vi "Sensor Reads.vi"() -> ()   [LabVIEW 2017]
uses:
  Refnum Names.vi
  <vilib>/Rock Robotics/Network Tables/NT Write Boolean.vi
  Lift/Lift Globals.vi
  <vilib>/Rock Robotics/WPI/ThirdParty/Phoenix-LabVIEW/Motor Controller/Get/CTRE_Phoenix_MotorController_GetSelectedSensorData.vi
  <vilib>/Rock Robotics/Network Tables/NT Write Number.vi
  Intake/Intake Globals.vi
  Intake Rotation/Intake Rotation Globals.vi
  <vilib>/Rock Robotics/WPI/ThirdParty/Phoenix-LabVIEW/Pigeon IMU/CTRE_PigeonIMU_GetRawGyro.vi
  <vilib>/Rock Robotics/WPI/ThirdParty/Phoenix-LabVIEW/Pigeon IMU/CTRE_PigeonIMU_GetYPR.vi
  Drive/Drive Globals.vi
  <vilib>/Rock Robotics/Network Tables/NT Write String.vi
panel:
  out "Z":dbl
  out "Match Time":string
  out "Robot Distance":dbl
  out "Robot Heading":dbl
  out "Arm Position":i32
  out "Cube IR":bool
  out "Arm Upper Limit Switch":bool
  out "Arm Lower Limit Switch":bool
  out "Lift Upper Switch":bool
  out "Lift Lower Switch":bool
  out "Lift Position":i32
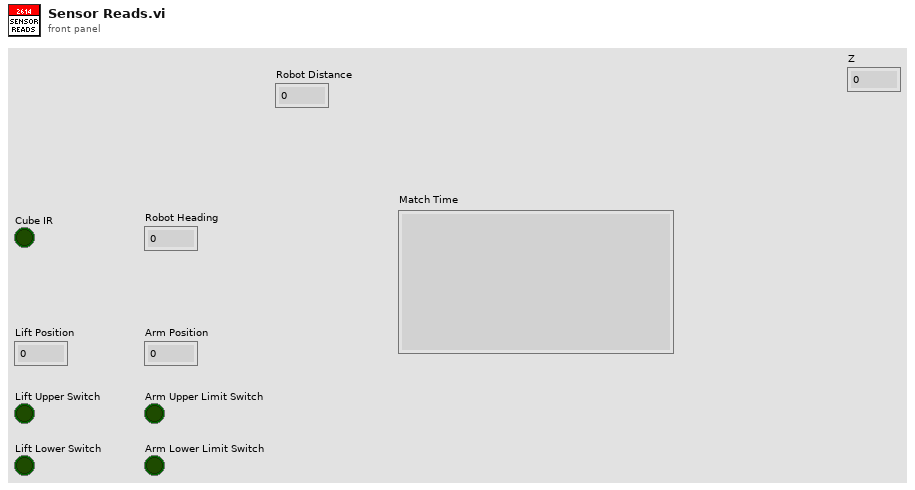
[diagram p1: front panel]
types:
  T1 = typedef "WPI_SwitchDevRef.ctl" = cluster{"DevStatus":errorcluster, "DIO Channel":T2, "CntIndex":T3, "Normally Closed":bool}
  T2 = typedef "FPGA_DIOChannel.ctl" = enum8{"DIO 0", "DIO 1", "DIO 2", "DIO 3", "DIO 4", "DIO 5", "DIO 6", "DIO 7", "DIO 8", "DIO 9", "DIO MXP 0", "DIO MXP 1", "DIO MXP 2", "DIO MXP 3", "DIO MXP 4", "DIO MXP 5", "DIO MXP 6", "DIO MXP 7", "DIO MXP 8", "DIO MXP 9", "DIO MXP 10", "DIO MXP 11", "DIO MXP 12", "DIO MXP 13", "DIO MXP 14", "DIO MXP 15", "SPI Port CS1", "SPI Port CS2", "SPI Port CS3", "SPI Port MISO", "SPI Port MOSI", "Invalid"}
  T3 = typedef "FPGA_CounterCtrSystemIndex.ctl" = enum8{"Ctr 0", "Ctr 1", "Ctr 2", "Ctr 3", "Ctr 4", "Ctr 5", "Ctr 6", "Ctr 7", "Invalid"}
  T4 = typedef "WPI_MotorControlDeviceRef.ctl" = cluster{"DeviceStatus":errorcluster, "Type":T5, "PWM":cluster{"PWM Channel":T6, "DeadBand":T7}, "CAN":cluster{"Device Number":u8, "SetOutput VI Ref":variant, "GetOutput VI Ref":variant, "Enable VI Ref":variant, "Disable VI Ref":variant, "Data":variant}, "Invert":bool, "DIO PWM":cluster{"PWM \"Enable\" Channel":T6, "DIOChannel":T2, "PWM Rate":dbl}}
  T5 = typedef "WPI_MotorControlType.ctl" = enum16{"PWM", "CAN", "DIO PWM"}
  T6 = typedef "FPGA_DIOPWMChannel.ctl" = enum8{"PWM 0", "PWM 1", "PWM 2", "PWM 3", "PWM 4", "PWM 5", "PWM 6", "PWM 7", "PWM 8", "PWM 9", "PWM MXP 0", "PWM MXP 1", "PWM MXP 2", "PWM MXP 3", "PWM MXP 4", "PWM MXP 5", "PWM MXP 6", "PWM MXP 7", "PWM MXP 8", "PWM MXP 9", "Invalid"}
  T7 = typedef "WPI_PWMDeadband.ctl" = cluster{"Name":string, "maxPositivePwm":i32, "minPositivePwm":i32, "centerPwm":i32, "maxNegativePwm":i32, "minNegativePwm":i32, "angularRange":u16}
  T8 = typedef "WPI_DigitalInputDevRef.ctl" = cluster{"DevStatus":errorcluster, "DIO Channel":T2}
  T9 = typedef "CTRE_PigeonIMU_DeviceRef.ctl" = cluster{"DeviceStatus":errorcluster, "Device Number":u8, "Type":T10, "Device ID":u32, "Handle":u64, "UsageFrame":u32, "Library Path":path}
  T10 = typedef "CTRE_PigeonIMU_ConnectionType.ctl" = u32
  T11 = cluster{"X":dbl, "Y":dbl, "Z":dbl, "Magnitude":dbl}
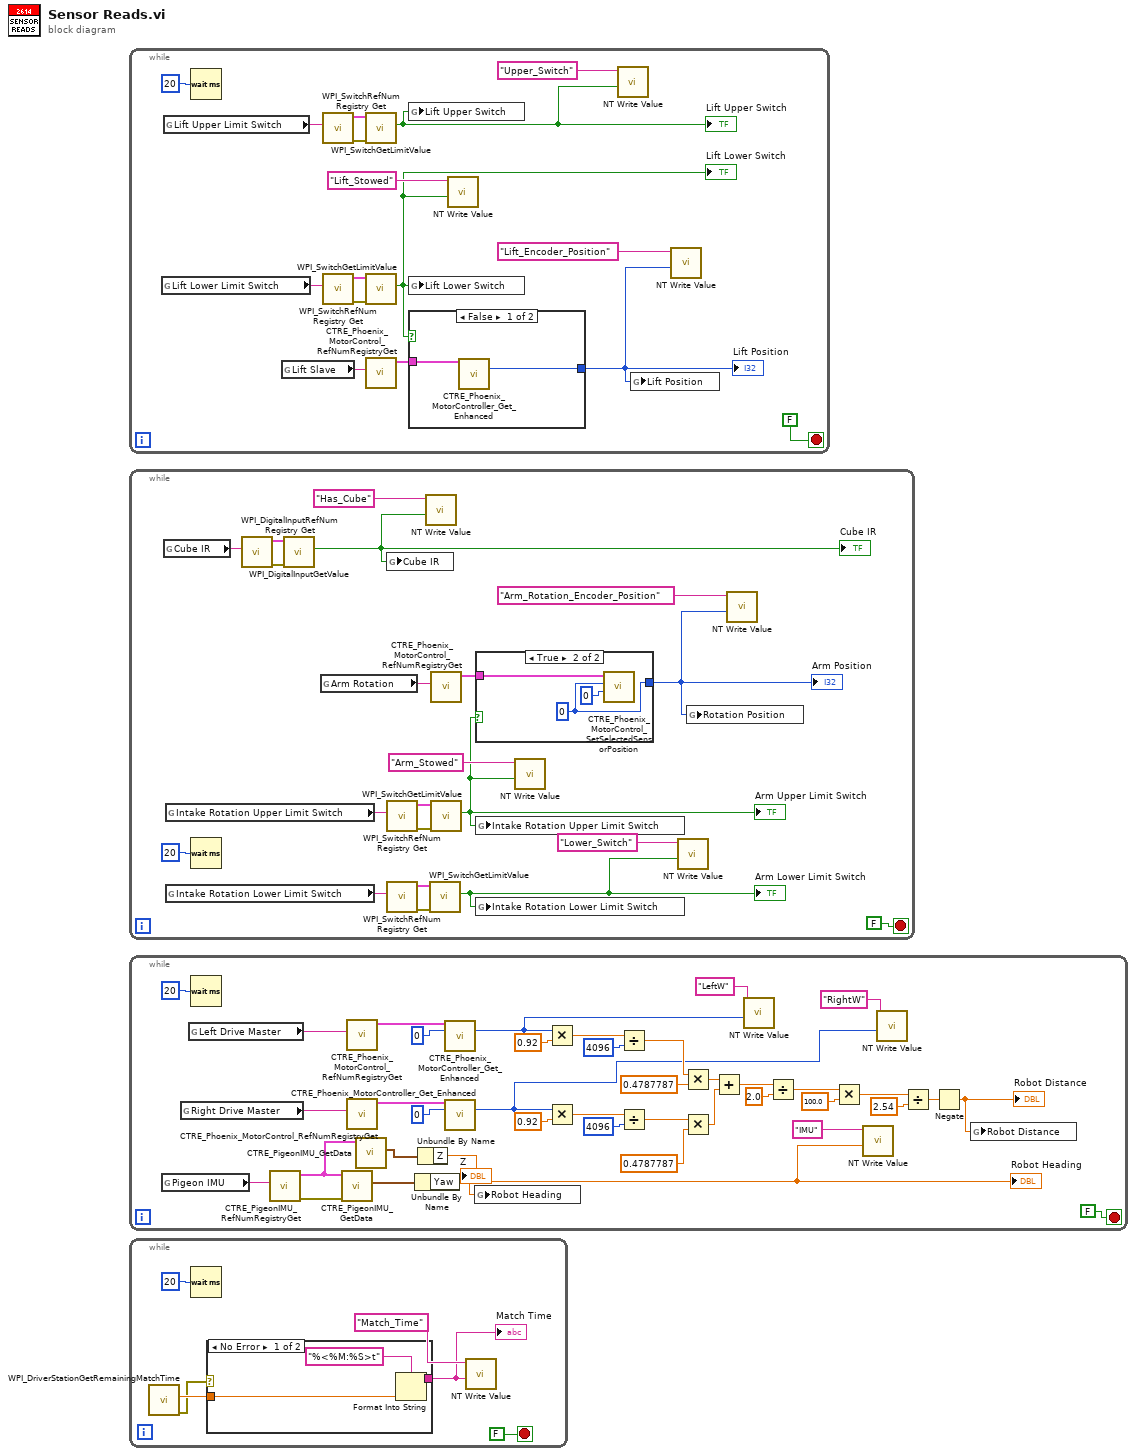
[diagram p0: block diagram]
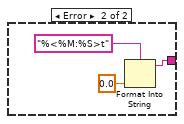
[diagram p2: hidden frame]
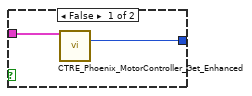
[diagram p3: hidden frame]
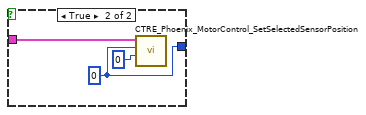
[diagram p4: hidden frame]
diagram:
  n1 = while {
    stop <- FALSE stop-if-true
    n2 = global read "Refnum Names.vi" "Lift Lower Limit Switch"() -> (w11:string)
    n3 = global read "Refnum Names.vi" "Lift Upper Limit Switch"() -> (w12:string)
    n4 = Wait (ms)(milliseconds to wait=u32 20) -> ()  [unwired: 1 out]
    n5 = global read "Refnum Names.vi" "Lift Slave"() -> (w8:string)
    n6 = call <vilib>:"WPI_SwitchRefNum Registry Get.vi"("refnum name"=w12) -> ("error out"=w13:errorcluster, "SwitchDevRef"=w14:T1)  [unwired: 9 in]
    n7 = call <vilib>:"WPI_SwitchRefNum Registry Get.vi"("refnum name"=w11) -> ("error out"=w10:errorcluster, "SwitchDevRef"=w9:T1)  [unwired: 9 in]
    n8 = call <vilib>:"WPI_SwitchGetLimitValue.vi"("error in (no error)"=w13, "SwitchDevRef"=w14) -> ("Switch Pressed"=w2:bool)  [unwired: 7 in, 2 out]
    "Lift Upper Switch" <- w2
    n9 = call <vilib>:"WPI_SwitchGetLimitValue.vi"("error in (no error)"=w10, "SwitchDevRef"=w9) -> ("Switch Pressed"=w5:bool)  [unwired: 7 in, 2 out]
    "Lift Lower Switch" <- w5
    n10 = call <vilib>:"CTRE_Phoenix_MotorControl_RefNumRegistryGet.vi"("refnum name"=w8) -> ("PhoenixMotorControlDevRef"=w7:T4)  [unwired: 9 in, 1 out]
    n11 = global write "Lift Globals.vi" "Lift Upper Switch"(w2) -> ()
    n12 = global write "Lift Globals.vi" "Lift Lower Switch"(w5) -> ()
    n13 = case shown="False" w5 {
      tunnel: w7 -> [w18 w21]
      tunnel: [w17 w19] -> w3
      frame False {
        n14 = call-poly <vilib>:"CTRE_Phoenix_MotorController_Get_Enhanced.vi"("PhoenixMotorControlDevRef"=w18) -> ("Position (Raw Sensor Units)"=w17:i32)  [unwired: 11 in, 3 out]
      }
      frame True {
        w19 = 0 ("New Sensor Position")
        n15 = call <vilib>:"CTRE_Phoenix_MotorControl_SetSelectedSensorPosition.vi"("pidLoopIdx"=u32 0, "New Sensor Position"=w19, "PhoenixMotorControlDevRef"=w21) -> ()  [unwired: 7 in, 2 out]
      }
    }
    "Lift Position" <- w3
    n16 = call-poly <vilib>:"NT Write Value.vi"("Boolean"=w5, "Name"="Lift_Stowed") -> ()  [unwired: 9 in, 1 out]
    n17 = call-poly <vilib>:"NT Write Value.vi"("Boolean"=w2, "Name"="Upper_Switch") -> ()  [unwired: 9 in, 1 out]
    n18 = global write "Lift Globals.vi" "Lift Position"(w3) -> ()
    n19 = call-poly <vilib>:"NT Write Value.vi"("Numeric"=w3, "Name"="Lift_Encoder_Position") -> ()  [unwired: 9 in, 1 out]
  }
  n20 = while {
    stop <- FALSE stop-if-true
    n21 = global read "Refnum Names.vi" "Cube IR"() -> (w40:string)
    n22 = global read "Refnum Names.vi" "Intake Rotation Upper Limit Switch"() -> (w37:string)
    n23 = global read "Refnum Names.vi" "Intake Rotation Lower Limit Switch"() -> (w36:string)
    n24 = Wait (ms)(milliseconds to wait=u32 20) -> ()  [unwired: 1 out]
    n25 = call <vilib>:"WPI_DigitalInputRefNum Registry Get.vi"("refnum name"=w40) -> ("error out"=w39:errorcluster, "DigitalInputDevRef"=w38:T8)  [unwired: 9 in]
    n26 = call <vilib>:"WPI_DigitalInputGetValue.vi"("error in (no error)"=w39, "DigitalInputDevRef"=w38) -> ("Value"=w26:bool)  [unwired: 7 in, 2 out]
    "Cube IR" <- w26
    n27 = global read "Refnum Names.vi" "Arm Rotation"() -> (w31:string)
    n28 = global write "Intake Globals.vi" "Cube IR"(w26) -> ()
    n29 = call <vilib>:"WPI_SwitchRefNum Registry Get.vi"("refnum name"=w37) -> ("error out"=w33:errorcluster, "SwitchDevRef"=w32:T1)  [unwired: 9 in]
    n30 = call <vilib>:"WPI_SwitchRefNum Registry Get.vi"("refnum name"=w36) -> ("error out"=w34:errorcluster, "SwitchDevRef"=w35:T1)  [unwired: 9 in]
    n31 = call-poly <vilib>:"NT Write Value.vi"("Boolean"=w26, "Name"="Has_Cube") -> ()  [unwired: 9 in, 1 out]
    n32 = call <vilib>:"WPI_SwitchGetLimitValue.vi"("error in (no error)"=w34, "SwitchDevRef"=w35) -> ("Switch Pressed"=w23:bool)  [unwired: 7 in, 2 out]
    "Arm Lower Limit Switch" <- w23
    n33 = call <vilib>:"CTRE_Phoenix_MotorControl_RefNumRegistryGet.vi"("refnum name"=w31) -> ("PhoenixMotorControlDevRef"=w30:T4)  [unwired: 9 in, 1 out]
    n34 = call <vilib>:"WPI_SwitchGetLimitValue.vi"("error in (no error)"=w33, "SwitchDevRef"=w32) -> ("Switch Pressed"=w24:bool)  [unwired: 7 in, 2 out]
    "Arm Upper Limit Switch" <- w24
    n35 = case shown="True" w24 {
      tunnel: [w44 w46] -> w27
      tunnel: w30 -> [w43 w45]
      frame False {
        n36 = call-poly <vilib>:"CTRE_Phoenix_MotorController_Get_Enhanced.vi"("PhoenixMotorControlDevRef"=w43) -> ("Position (Raw Sensor Units)"=w44:i32)  [unwired: 11 in, 3 out]
      }
      frame True {
        w46 = 0 ("New Sensor Position")
        n37 = call <vilib>:"CTRE_Phoenix_MotorControl_SetSelectedSensorPosition.vi"("pidLoopIdx"=u32 0, "New Sensor Position"=w46, "PhoenixMotorControlDevRef"=w45) -> ()  [unwired: 7 in, 2 out]
      }
    }
    "Arm Position" <- w27
    n38 = global write "Intake Rotation Globals.vi" "Intake Rotation Upper Limit Switch"(w24) -> ()
    n39 = global write "Intake Rotation Globals.vi" "Intake Rotation Lower Limit Switch"(w23) -> ()
    n40 = call-poly <vilib>:"NT Write Value.vi"("Boolean"=w24, "Name"="Arm_Stowed") -> ()  [unwired: 9 in, 1 out]
    n41 = call-poly <vilib>:"NT Write Value.vi"("Boolean"=w23, "Name"="Lower_Switch") -> ()  [unwired: 9 in, 1 out]
    n42 = global write "Intake Rotation Globals.vi" "Rotation Position"(w27) -> ()
    n43 = call-poly <vilib>:"NT Write Value.vi"("Numeric"=w27, "Name"="Arm_Rotation_Encoder_Position") -> ()  [unwired: 9 in, 1 out]
  }
  n44 = while {
    stop <- FALSE stop-if-true
    n45 = global read "Refnum Names.vi" "Pigeon IMU"() -> (w85:string)
    n46 = global read "Refnum Names.vi" "Right Drive Master"() -> (w82:string)
    n47 = global read "Refnum Names.vi" "Left Drive Master"() -> (w81:string)
    n48 = Wait (ms)(milliseconds to wait=u32 20) -> ()  [unwired: 1 out]
    n49 = call <vilib>:"CTRE_PigeonIMU_RefNumRegistryGet.vi"("refnum name"=w85) -> ("error out"=w84:errorcluster, "PigeonIMUDevRef"=w49:T9)  [unwired: 9 in]
    n50 = call-poly <vilib>:"CTRE_PigeonIMU_GetData.vi"("error in (no error)"=w84, "PigeonIMUDevRef"=w49) -> ("Yaw Pitch Roll"=w83:cluster{"Yaw":dbl, "Pitch":dbl, "Roll":dbl})  [unwired: 7 in, 2 out]
    n51 = call <vilib>:"CTRE_Phoenix_MotorControl_RefNumRegistryGet.vi"("refnum name"=w81) -> ("PhoenixMotorControlDevRef"=w77:T4)  [unwired: 9 in, 1 out]
    n52 = call <vilib>:"CTRE_Phoenix_MotorControl_RefNumRegistryGet.vi"("refnum name"=w82) -> ("PhoenixMotorControlDevRef"=w80:T4)  [unwired: 9 in, 1 out]
    n53 = call-poly <vilib>:"CTRE_PigeonIMU_GetData.vi"("PigeonIMUDevRef"=w49) -> ("Gyro DPS"=w50:T11)  [unwired: 8 in, 2 out]
    n54 = Unbundle By Name(w83) -> ("Yaw"=w51:dbl)
    "Robot Heading" <- w51
    n55 = Unbundle By Name(w50) -> ("Z"=→"Z":dbl)
    n56 = call-poly <vilib>:"CTRE_Phoenix_MotorController_Get_Enhanced.vi"("PhoenixMotorControlDevRef"=w77, "pidLoopIdx"=u32 0) -> ("Position (Raw Sensor Units)"=w55:i32)  [unwired: 10 in, 3 out]
    n57 = call-poly <vilib>:"CTRE_Phoenix_MotorController_Get_Enhanced.vi"("PhoenixMotorControlDevRef"=w80, "pidLoopIdx"=u32 0) -> ("Position (Raw Sensor Units)"=w52:i32)  [unwired: 10 in, 3 out]
    n58 = global write "Drive Globals.vi" "Robot Heading"(w51) -> ()
    n59 = Multiply(x=w55, y=0.92) -> (x*y=w69:dbl)
    n60 = Multiply(x=w52, y=0.92) -> (x*y=w70:dbl)
    n61 = Divide(x=w69, y=4096) -> (x/y=w73:dbl)
    n62 = Divide(x=w70, y=4096) -> (x/y=w74:dbl)
    n63 = Multiply(x=w73, y=0.4787787) -> (x*y=w66:dbl)
    n64 = Multiply(x=w74, y=0.4787787) -> (x*y=w65:dbl)
    n65 = Add(x=w66, y=w65) -> (x+y=w64:dbl)
    n66 = call-poly <vilib>:"NT Write Value.vi"("Numeric"=w55, "Name"="LeftW") -> ()  [unwired: 9 in, 1 out]
    n67 = Divide(x=w64, y=2.0) -> (x/y=w62:dbl)
    n68 = Multiply(x=w62, y=100.0) -> (x*y=w60:dbl)
    n69 = call-poly <vilib>:"NT Write Value.vi"("Numeric"=w51, "Name"="IMU") -> ()  [unwired: 9 in, 1 out]
    n70 = call-poly <vilib>:"NT Write Value.vi"("Numeric"=w52, "Name"="RightW") -> ()  [unwired: 9 in, 1 out]
    n71 = Divide(x=w60, y=2.54) -> (x/y=w58:dbl)
    n72 = Negate(x=w58) -> (-x=w57:dbl)
    "Robot Distance" <- w57
    n73 = global write "Drive Globals.vi" "Robot Distance"(w57) -> ()
  }
  n74 = while {
    stop <- FALSE stop-if-true
    n75 = call <vilib>:"WPI_DriverStationGetRemainingMatchTime.vi"() -> ("error out"=w88:errorcluster, "Match Time(s)"=w91:sgl)  [unwired: 10 in]
    n76 = Wait (ms)(milliseconds to wait=u32 20) -> ()  [unwired: 1 out]
    n77 = case shown="No Error" w88 {
      tunnel: w91 -> [w96 _]
      tunnel: [w94 w99] -> w89
      frame No Error {
        n78 = Format Into String(format string="%<%M:%S>t", w96) -> (resulting string=w94:string)  [unwired: 2 in, 1 out]
      }
      frame Error {
        n79 = Format Into String(format string="%<%M:%S>t", sgl 0.0 ("input 1")) -> (resulting string=w99:string)  [unwired: 2 in, 1 out]
      }
    }
    "Match Time" <- w89
    n80 = call-poly <vilib>:"NT Write Value.vi"("String"=w89, "Name"="Match_Time") -> ()  [unwired: 9 in, 1 out]
  }
